vi "FTW-TestExecutive-Results-Serialize.vi"(0 "Results":T1 {"Start Time" format="%<%Y-%m-%d %H:%M:%S%03u>T"; "Elapsed Time" format="%<%H:%M:%S%3u>t"}, 11 "error in (no error)":errorcluster) -> (4 "Serialized Results":string, 15 "error out":errorcluster)   [LabVIEW 2015]
doc: "This VI is intended to be used <b>only by test steps</b> to report their results to the Test Executive"
uses:
  FTW-TestExecutive-Results.ctl
  container/FTW-Container.lvclass
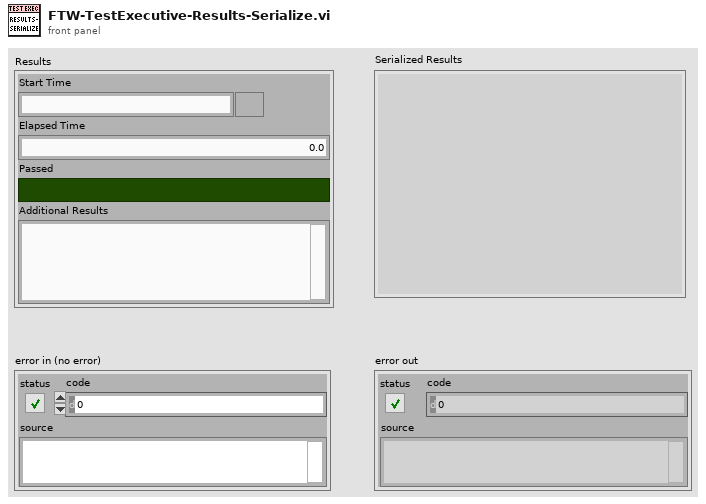
[diagram p1: front panel]
types:
  T1 = typedef "FTW-TestExecutive-Results.ctl" = cluster{"Start Time":timestamp, "Elapsed Time":dbl, "Passed":bool, "Additional Results":string}
  T2 = typedef "FTW-JSON-Type.ctl" = enum8{"Not Found", "Object", "Array", "String", "Number", "Boolean", "null"}
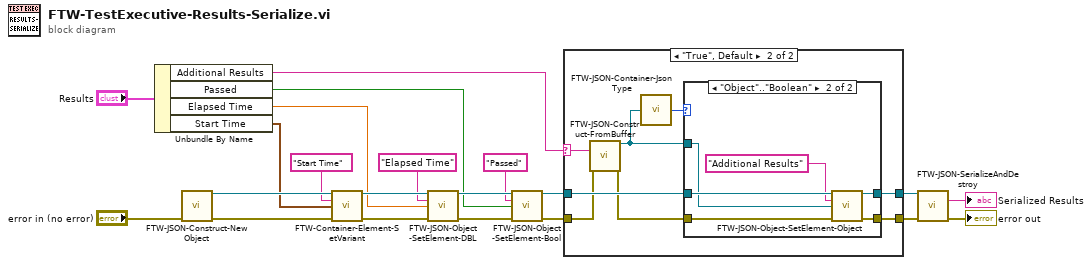
[diagram p0: block diagram]
diagram:
  n1 = Unbundle By Name("Results") -> ("Additional Results"=w14:string, "Passed"=w3:bool, "Elapsed Time"=w2:dbl, "Start Time"=w1:timestamp)
  n2 = call "FTW-JSON-Construct-NewObject.vi"("error in"="error in (no error)") -> ("JSON"=w12:refnum<class "FTW-Container.lvclass">, "error out"=w16:errorcluster)  [unwired: 13 in]
  n3 = call "FTW-Container-Element-SetVariant.vi"("FTW-Container In"=w12, "Element Name"="Start Time", "Variant"=w1, "error in"=w16) -> ("FTW-Container Out"=w9:refnum<class "FTW-Container.lvclass">, "error out"=w13:errorcluster)  [unwired: 9 in, 1 out]
  n4 = call "FTW-JSON-Object-SetElement-DBL.vi"("JSON"=w9, "Key"="Elapsed Time" ("Element Name"), "Value"=w2, "error in"=w13) -> ("JSON out"=w7:refnum<class "FTW-Container.lvclass">, "error out"=w10:errorcluster)  [unwired: 10 in]
  n5 = call "FTW-JSON-Object-SetElement-Bool.vi"("JSON"=w7, "Key"="Passed" ("Element Name"), "Value"=w3, "error in"=w10) -> ("JSON out"=w6:refnum<class "FTW-Container.lvclass">, "error out"=w8:errorcluster)  [unwired: 10 in]
  n6 = case shown="\"True\", Default" w14 {
    selector: w14 -> [_ w29]
    tunnel: [w22 w31] -> w20
    tunnel: w6 -> [w23 w30]
    tunnel: [w23 w27] -> w17
    tunnel: w8 -> [w22 w26]
    frame "" {
    }
    frame "True", Default {
      n7 = call "FTW-JSON-Construct-FromBuffer.vi"("JSON String (UTF-8)"=w29, "error in"=w26) -> ("JSON"=w24:refnum<class "FTW-Container.lvclass">, "error out"=w25:errorcluster)  [unwired: 12 in]
      n8 = call "FTW-JSON-Container-JsonType.vi"("Container"=w24) -> ("JSON Element Type"=w28:T2)  [unwired: 14 in]
      n9 = case shown="\"Object\"..\"Boolean\"" w28 {
        tunnel: w25 -> [w32 w39]
        tunnel: [w32 w38] -> w31
        tunnel: w30 -> [w33 w37]
        tunnel: [w33 w36] -> w27
        tunnel: w24 -> [_ w35]
        frame "Not Found", "null" {
        }
        frame "Object".."Boolean" {
          n10 = call "FTW-JSON-Object-SetElement-Object.vi"("JSON Object"=w37, "Key"="Additional Results", "JSON Sub-Object"=w35, "error in"=w39) -> ("JSON Root Object"=w36:refnum<class "FTW-Container.lvclass">, "error out"=w38:errorcluster)  [unwired: 10 in]
        }
      }
    }
  }
  n11 = call "FTW-JSON-SerializeAndDestroy.vi"("JSON"=w17, "error in"=w20) -> ("JSON String (UTF-8)"=→"Serialized Results":string, "error out"=→"error out":errorcluster)  [unwired: 12 in]
